vi "Error Handler for MHL and EHL.vi"(8 "ErrorIn":errorcluster, 9 "Ignore Errors":i32[](array[numeric]), 10 "Error MHL Name (\"Error\")":string="Error") -> (0 "ErrorOut":errorcluster)   [LabVIEW 2020, in "main.lvlib"]
doc: "Handle Errors in Message Loop"
uses:
  main.lvlib
panel:
  # "Description\n\nHandle Errors in Message Loop"
  # "INPUTS"
  # "OUTPUTS"
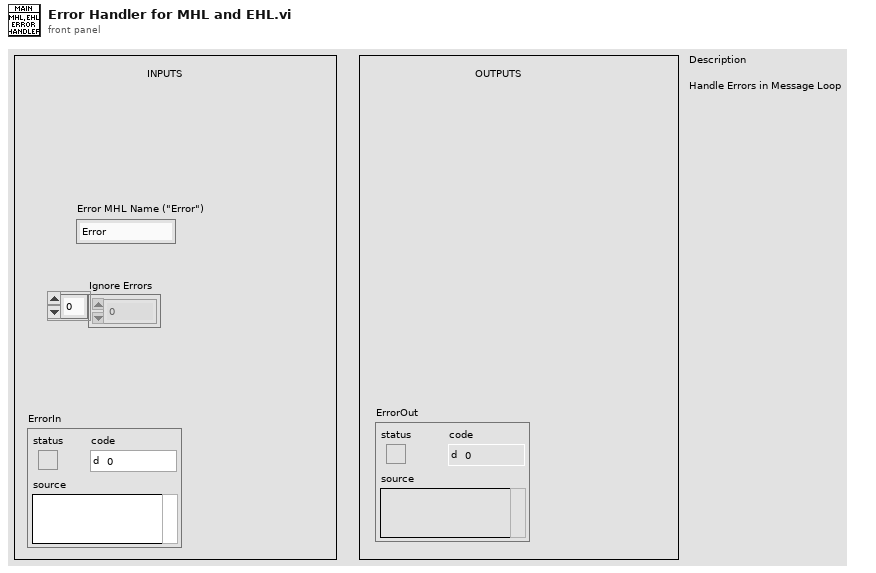
[diagram p1: front panel]
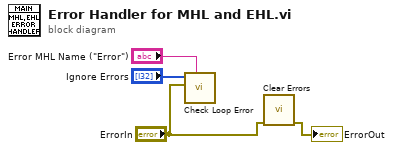
[diagram p0: block diagram]
diagram:
  n1 = call "Check Loop Error.vi"("Error MHL Name (\"Error\")"="Error MHL Name (\"Error\")", "ErrorIn"="ErrorIn", "Ignore Errors"="Ignore Errors") -> ()  [unwired: 8 in, 1 out]
  n2 = call <vilib>:"Clear Errors.vi"("error in (no error)"="ErrorIn") -> ("error out"=→"ErrorOut":errorcluster)  [unwired: 5 in, 1 out]
